vi "Execute Function.vi"(7 "Transmission Data Unit":refnum<class "Transmission Data Unit.lvclass">, 8 "error in":errorcluster, 10 "modbus request":refnum<class "Modbus Data Unit.lvclass">, 11 "Super Data Model in":refnum<class "Super Data Model.lvclass">) -> (0 "error out":errorcluster, 2 "modbus response":refnum<class "Modbus Data Unit.lvclass">, 3 "Super Data Model out":refnum<class "Super Data Model.lvclass">)   [LabVIEW 2013, in "Modbus Library - Advance.lvlib" / "Super Data Model.lvclass"]
uses:
  Super Data Model.lvclass
  Modbus Data Unit/Modbus Data Unit.lvclass
  Transmission Data Unit/Transmission Data Unit.lvclass
  Transmission Data Unit/Transmission Data Unit.lvclass/Transmission Data Unit.ctl
  Standard Data Model/Standard Data Model.lvclass
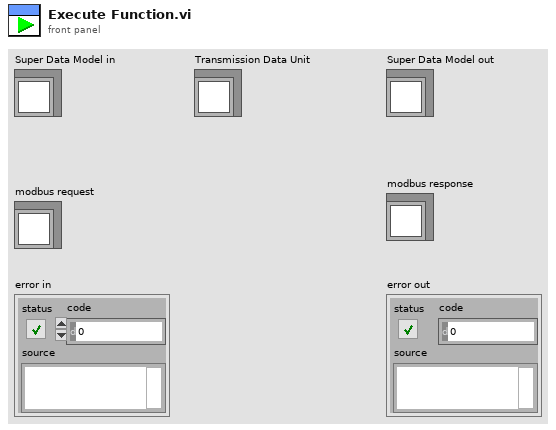
[diagram p1: front panel]
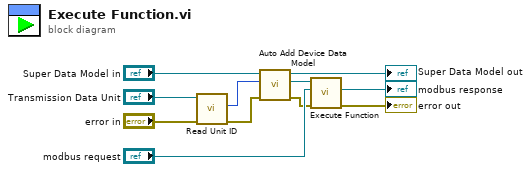
[diagram p0: block diagram]
diagram:
  n1 = call "Read Unit ID.vi"("error in"="error in", "transmission data unit in"="Transmission Data Unit") -> ("error out"=w5:errorcluster, "unit ID"=w7:u8)  [unwired: 7 in, 1 out]
  n2 = call "Auto Add Device Data Model.vi"("error in"=w5, "unit ID"=w7, "Super Data Model in"="Super Data Model in") -> ("error out"=w1:errorcluster, "device data model"=w3:refnum<class "Standard Data Model.lvclass">, "Super Data Model out"=→"Super Data Model out":refnum<class "Super Data Model.lvclass">)  [unwired: 6 in]
  n3 = call-dynamic "Execute Function.vi"("error in"=w1, "modbus request"="modbus request", "device data model in"=w3) -> ("error out"=→"error out":errorcluster, "modbus response"=→"modbus response":refnum<class "Modbus Data Unit.lvclass">)  [unwired: 6 in, 1 out]
